vi "FTW-Messenger-Construct.vi"(0 "Messenger Type":refnum<class "FTW-Messenger-Actor.lvclass">, 11 "error in":errorcluster) -> (4 "Actor Messenger":refnum<class "FTW-Messenger-Actor.lvclass">, 15 "error out":errorcluster)   [LabVIEW 2013, in "FTW-Messenger-Actor.lvclass"]
uses:
  FTW-Messenger-Actor.lvclass
  Message/FTW-Message.lvclass
  Messenger/FTW-Messenger.lvclass
  FTW-Messenger-Actor.lvclass/FTW-Messenger-Actor.ctl
panel:
  # "Inputs"
  # "Outputs"
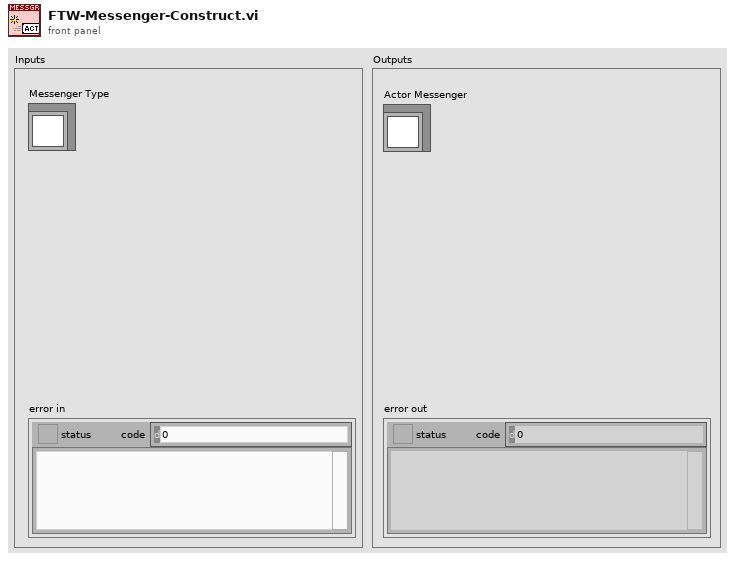
[diagram p1: front panel]
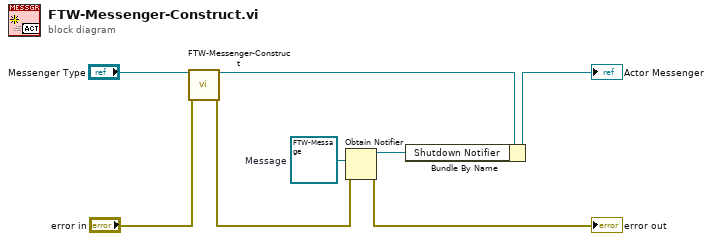
[diagram p0: block diagram]
diagram:
  w5 = refnum<class "FTW-Message.lvclass"> refnum  # Message
  n1 = call-parent "FTW-Messenger-Construct.vi"("Messenger Type"="Messenger Type", "error in"="error in") -> ("Messenger"=w7:refnum<class "FTW-Messenger-Actor.lvclass">, "error out"=w4:errorcluster)  [unwired: 12 in]
  n2 = Obtain Notifier(notification data type=w5, error in (no error)=w4) -> (notifier out=w1:refnum<notifier>, error out=→"error out":errorcluster)  [unwired: 2 in, 1 out]
  n3 = Bundle By Name(cluster=w7, "Shutdown Notifier"=w1) -> (→"Actor Messenger":refnum<class "FTW-Messenger-Actor.lvclass">)
